vi "sub_sebessegszamlalo.vi"(9 "Sebesseg":dbl(slide)=1.5254237288135593 scale=1.0..3.0, 10 "Szög":dbl(knob), 11 "Táv":dbl(slide) scale=0.0..1.2) -> (2 "Jobb":dbl(slide) scale=-5.0..5.0, 3 "Bal":dbl(slide) scale=-5.0..5.0 scale format="%0#1_1g")   [LabVIEW 2012]
panel:
  out "output variable":dbl format="%.2f"
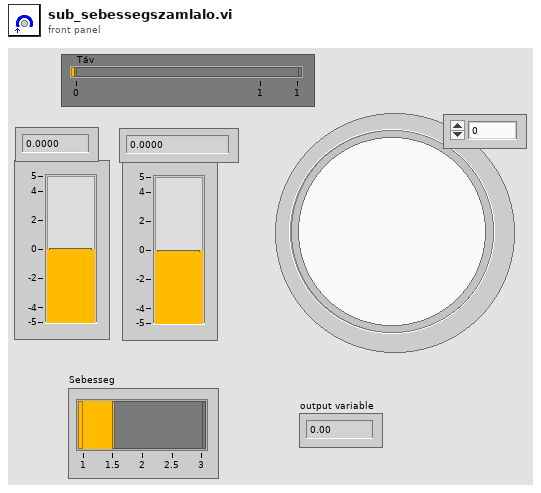
[diagram p1: front panel]
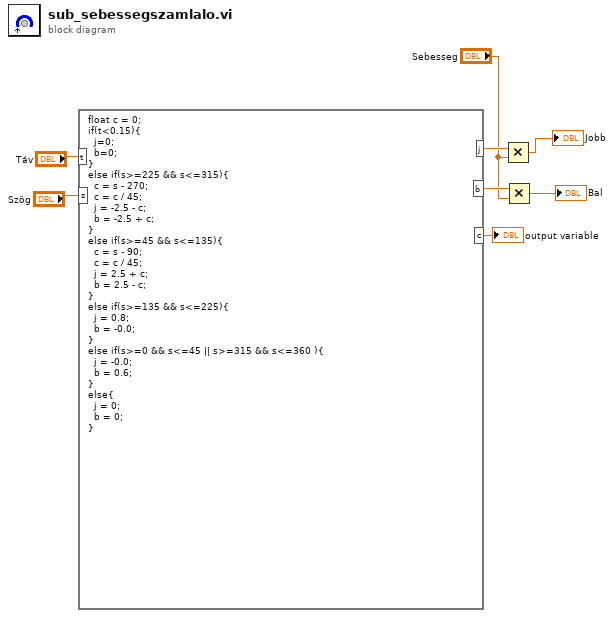
[diagram p0: block diagram]
diagram:
  n1 = formula code="float c = 0;\nif(t<0.15){\n  j=0; \n  b=0;\n}\nelse if(s>=225 && s<=315){\n  c = s - 270;\n  c = c / 45;\n  j = -2.5 - c;  \n  b = -2.5 + c;\n}\nelse if(s>=45 && s<=135){\n  c = s - 90;\n  c = c / 45;\n  j = 2.5 + c;  \n  b = 2.5 - c;\n}\nelse if(s>=135 && s<=225){\n  j = 0.8;  \n  b = -0.0;\n}\nelse if(s>=0 && s<=45 || s>=315 && s<=360 ){\n  j = -0.0;  \n  b = 0.6;\n}\nelse{\n  j = 0;\n  b = 0;\n}"("t"="Táv", "s"="Szög") -> ("j"=w6:dbl, "b"=w4:dbl, "c"=→"output variable":dbl)
  n2 = Multiply(x=w6, y="Sebesseg") -> (x*y=→"Jobb":dbl)
  n3 = Multiply(x=w4, y="Sebesseg") -> (x*y=→"Bal":dbl)
